vi "hardware_close_hardware.vi"(8 "error in (no error)":errorcluster, 11 "tt20 in":refnum<class "tt20.lvclass">) -> (0 "error out":errorcluster, 3 "tt20 out":refnum<class "tt20.lvclass">)   [LabVIEW 2015, in "tt20.lvclass"]
uses:
  tt20.lvclass
  tt20.lvclass/tt20.ctl
  C:/Users/MX-Microscope/Documents/LabVIEW Data/lvoop_campus_2018/Detector_Class/Swabian/time_tagger_vis/TTCSharp32.dll
  time_tagger_vis/TTCSharp32.dll
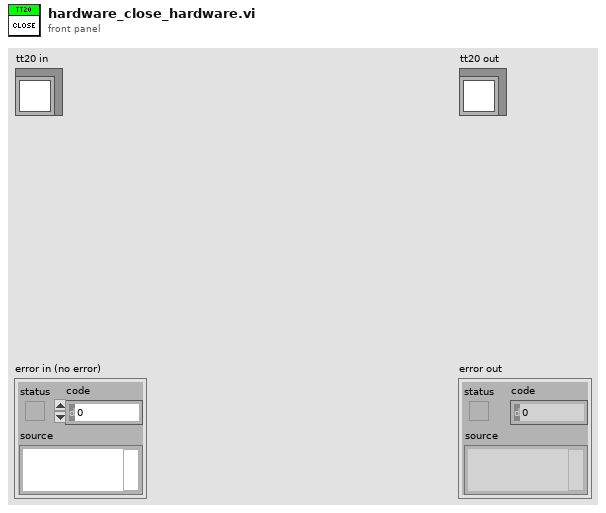
[diagram p1: front panel]
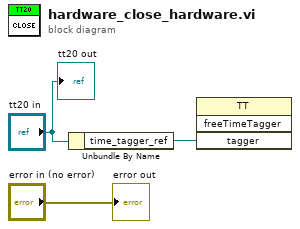
[diagram p0: block diagram]
diagram:
  n1 = Unbundle By Name("tt20 in") -> ("time_tagger_ref"=w2:refnum<k24>)
  n2 = invoke class="TT" method="freeTimeTagger"("tagger"=w2) -> ()  [unwired: 3 in, 4 out]
  "error out" <- "error in (no error)"
  "tt20 out" <- "tt20 in"
